vi "Offset (test).vi"(0 "RA offset":dbl format="%.2f", 1 "TCS control visa number":refnum<visa-resource-name>, 2 "TableVisaNumber":refnum<visa-resource-name>, 3 "InputVisaNumber":refnum<visa-resource-name> caption="PortNumber", 5 "DEC offset":dbl format="%.2f", 7 "Mode Offset":u32=4, 9 "Temps d'exposition":dbl=2.0 min=0.0 step=0.001 format="%.3f", 11 "Rot(rad)":dbl=3.635577729637803 format="%.2f", 12 "arcmin/pulse":dbl=5.367e-05 format="%.5e", 13 "RA Tel":dbl=45429.1344 caption="A. D." format="%<%H:%M:%S%1u>t", 14 "DEC Tel":dbl=164421.0216 caption="Déc." format="%<%H:%M:%S%0u>t") -> (8 "Undo offset":bool)   [LabVIEW 2010]
uses:
  Globals.vi
  Polymorphics/Distance(single).vi
panel:
  out "Error code":i8
  out "Guider was running":bool
  out "NewRA":dbl format="%.2f"
  out "NewDEC":dbl format="%.2f"
  out "Moffset":bool
  out "Goffset":bool=TRUE
  out "Undo startguide":bool
  in  "goto accel":u32=200 max=1000
  in  "goto vite":u32=30000 min=1 max=500000
  in  "goto lent":u32=200 min=1 max=500000
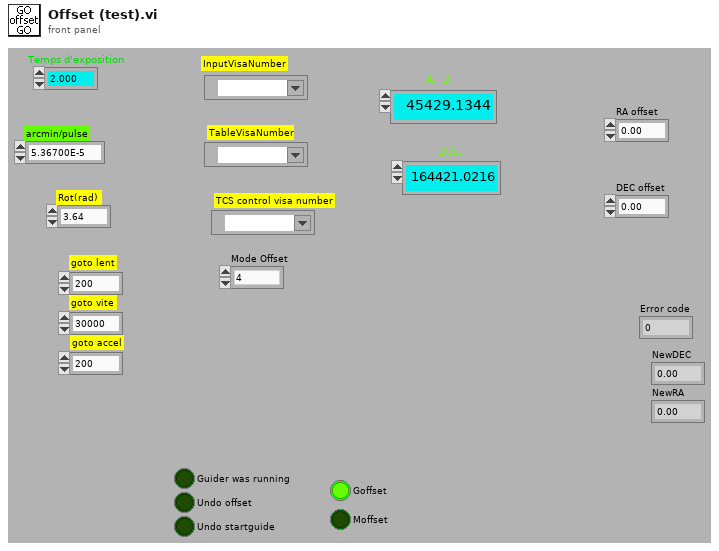
[diagram p1: front panel]
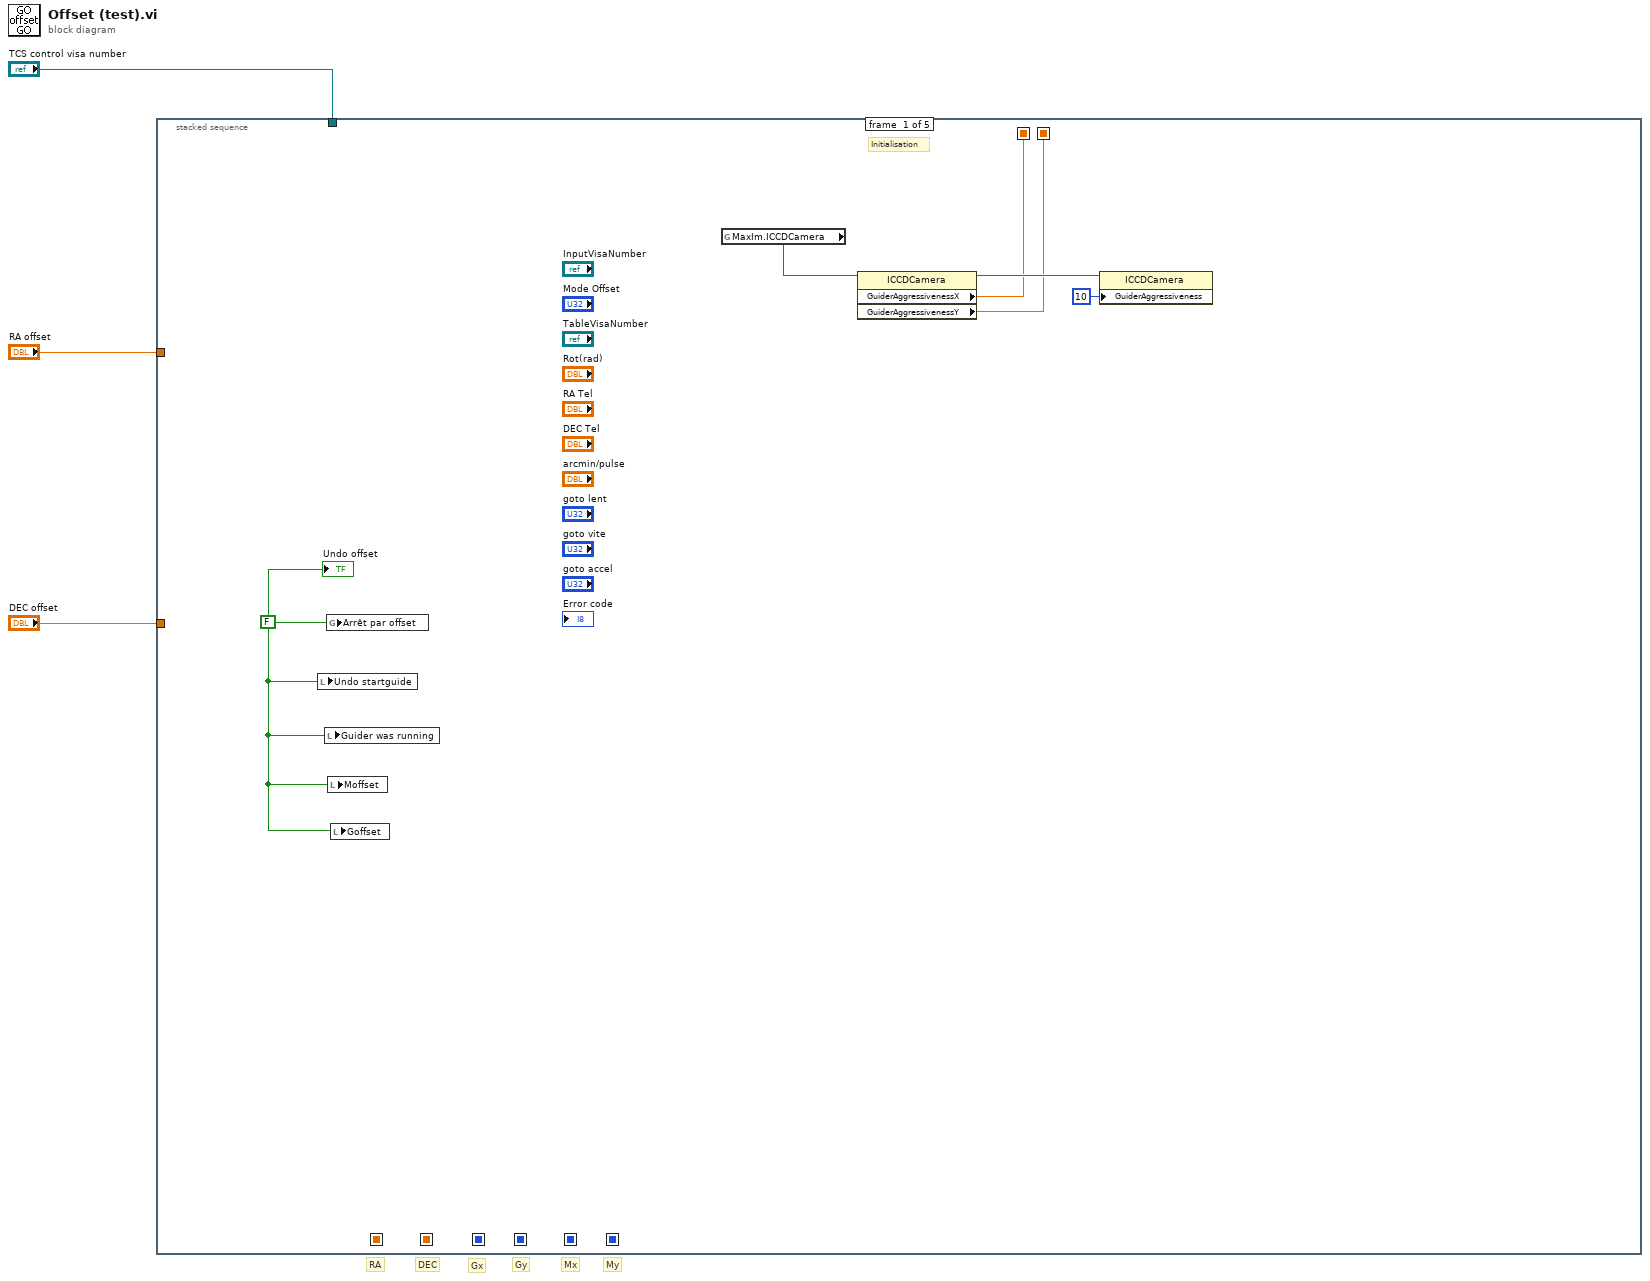
[diagram p0: block diagram]
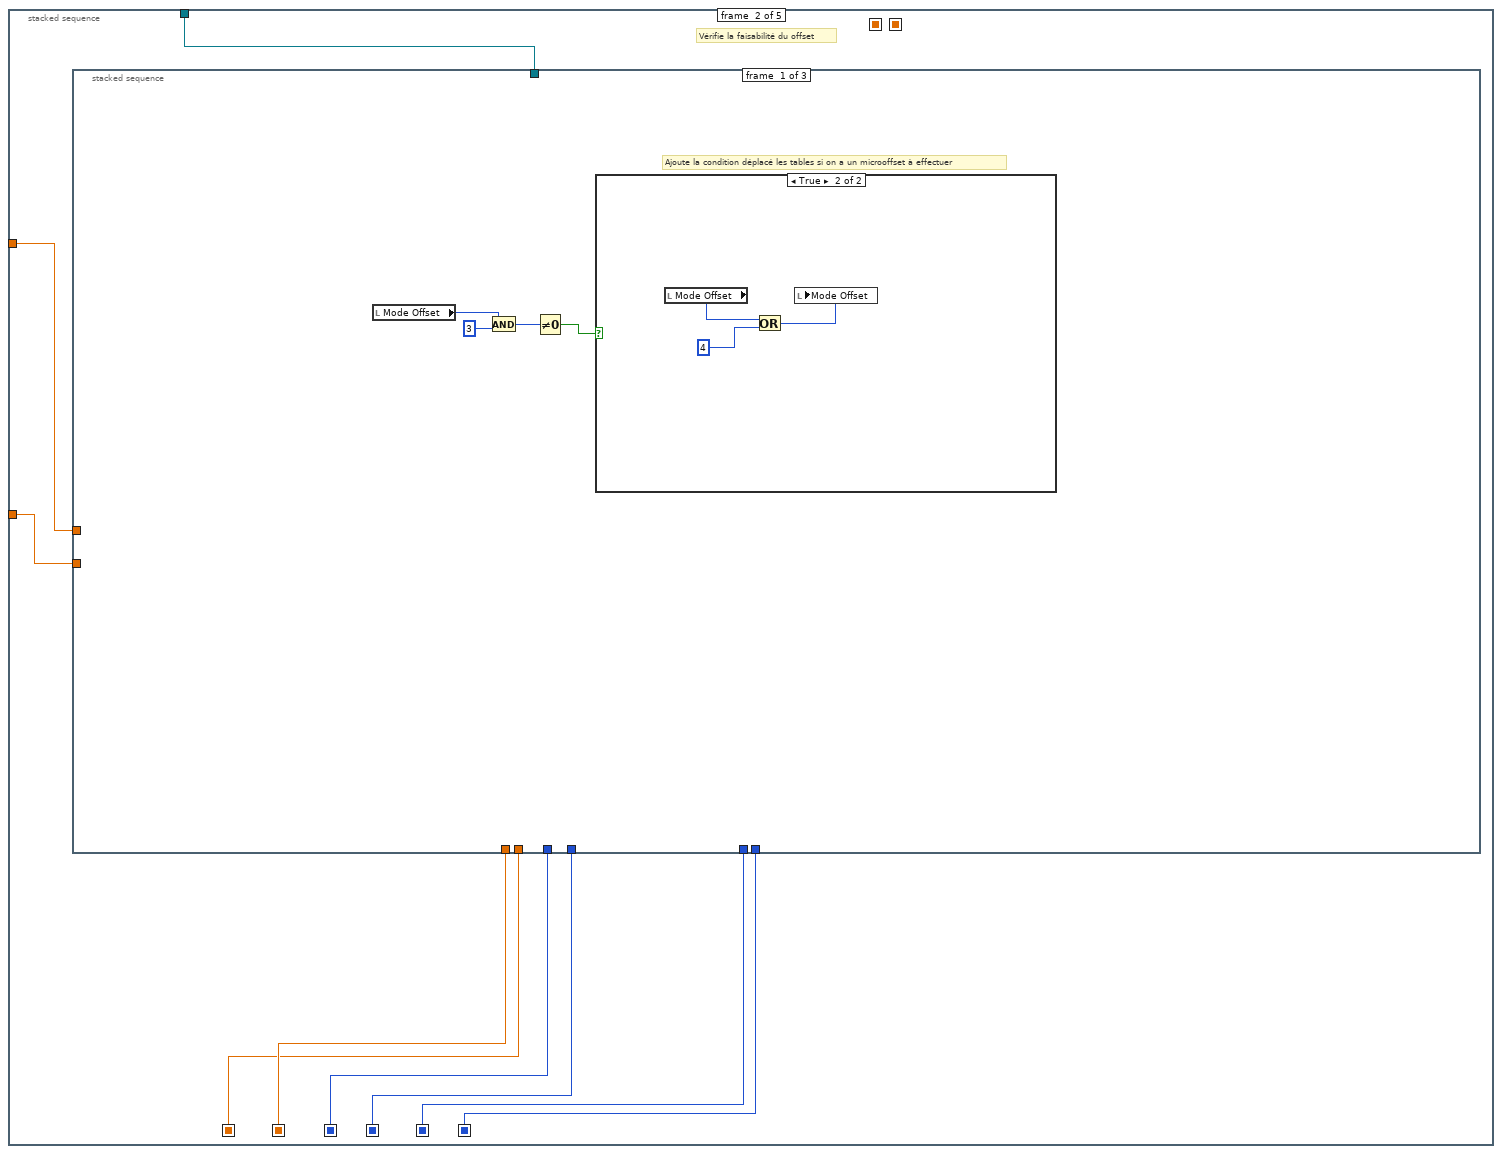
[diagram p2: hidden frame]
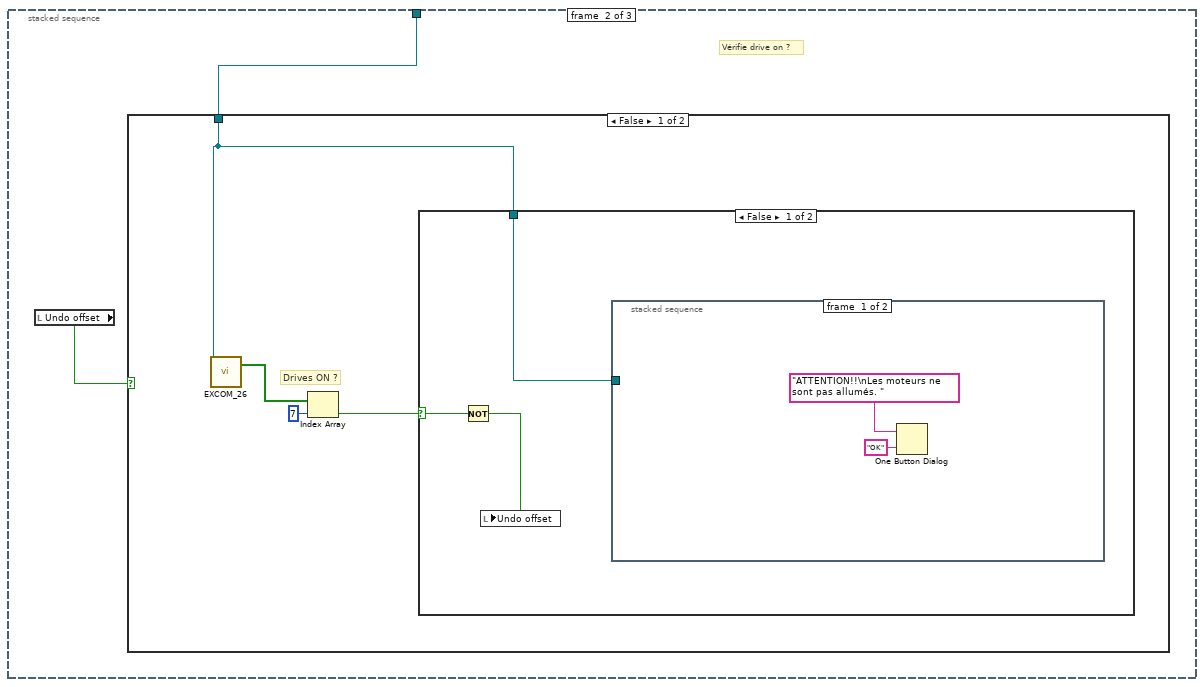
[diagram p4: hidden frame]
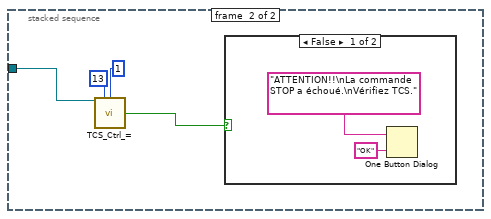
[diagram p5: hidden frame]
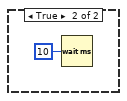
[diagram p6: hidden frame]
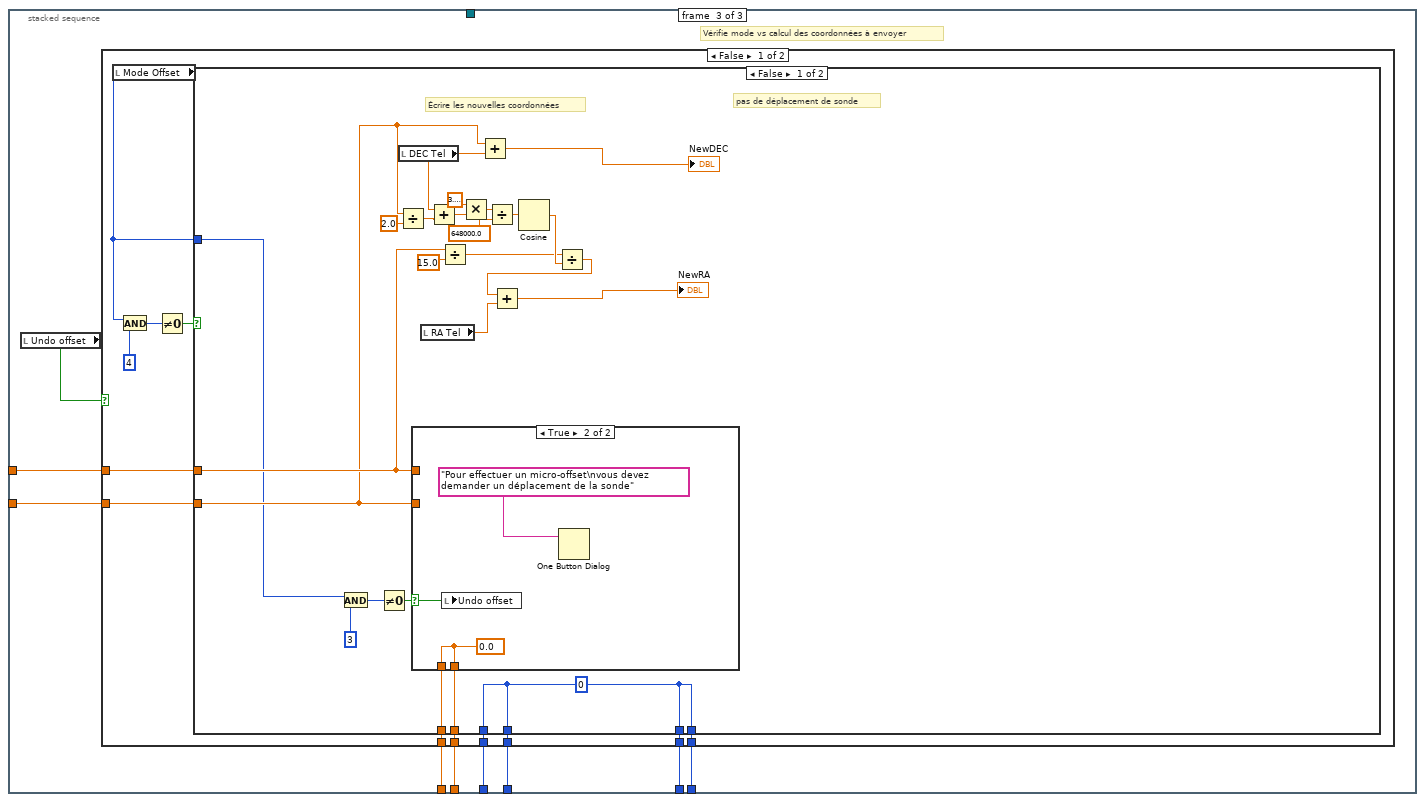
[diagram p9: hidden frame]
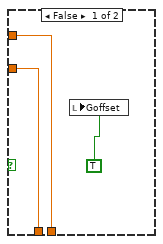
[diagram p10: hidden frame]
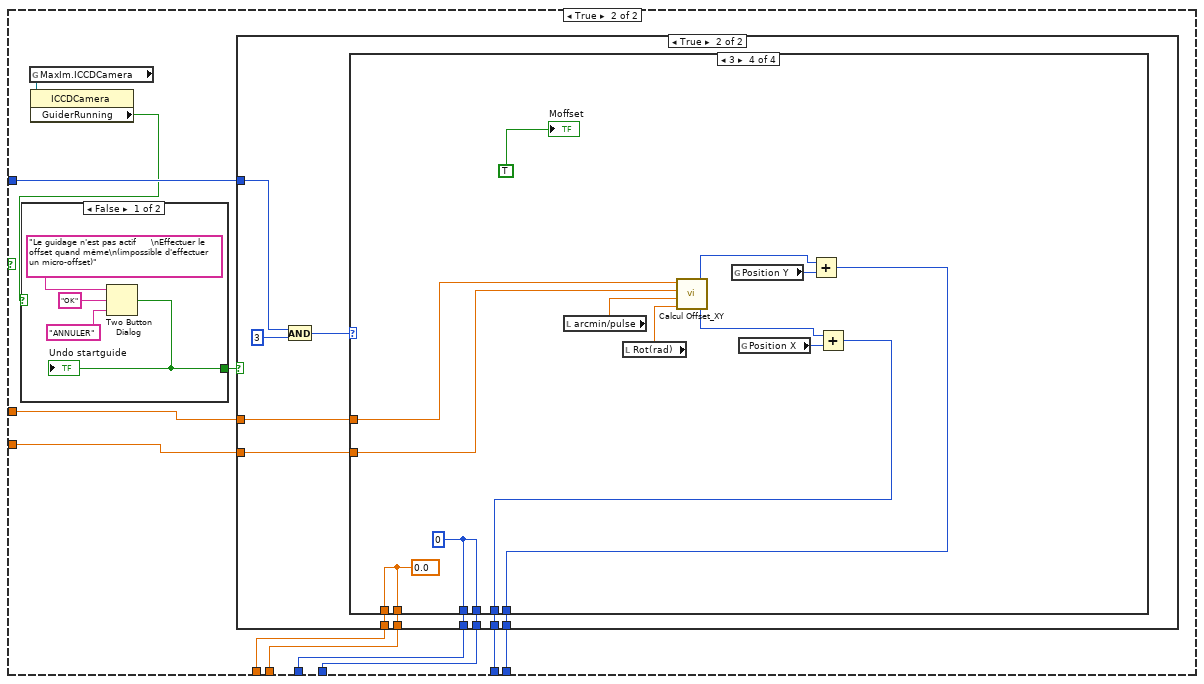
[diagram p11: hidden frame]
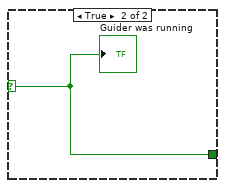
[diagram p12: hidden frame]
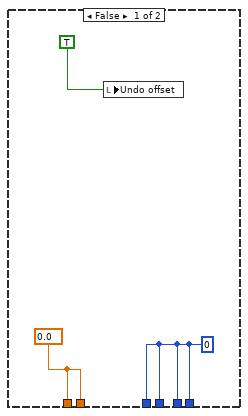
[diagram p13: hidden frame]
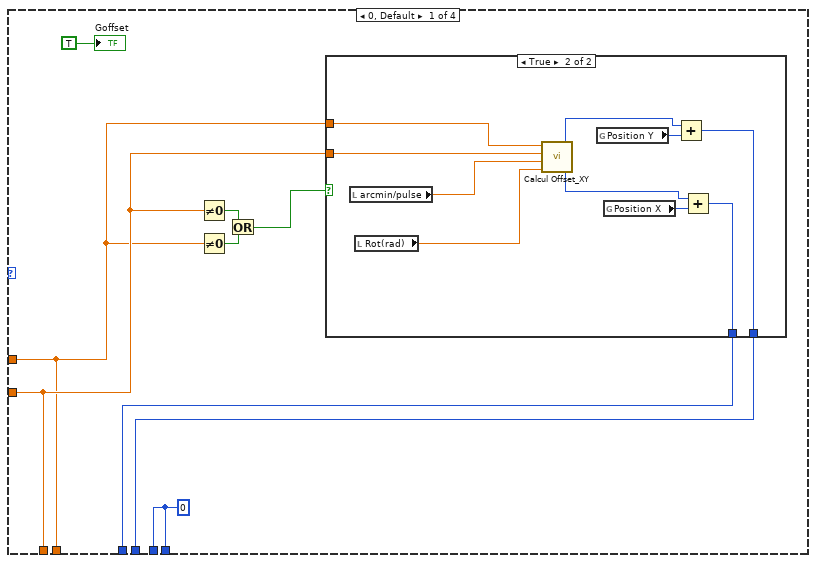
[diagram p14: hidden frame]
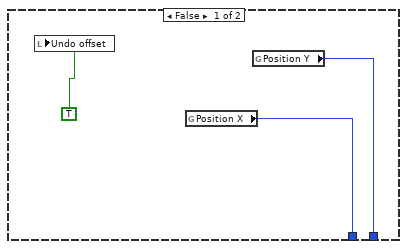
[diagram p15: hidden frame]
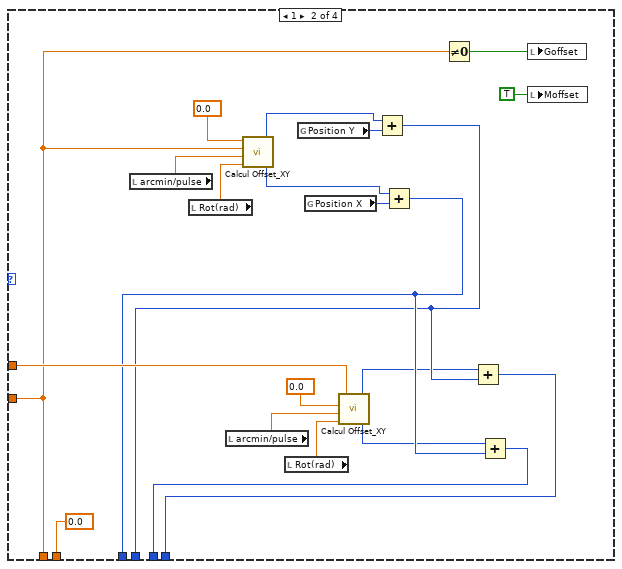
[diagram p16: hidden frame]
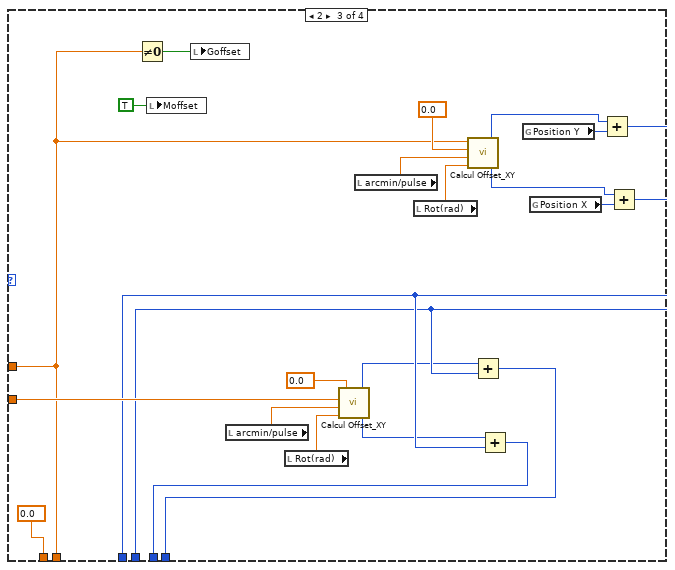
[diagram p17: hidden frame]
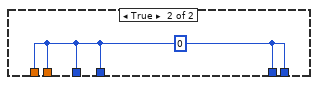
[diagram p18: hidden frame]
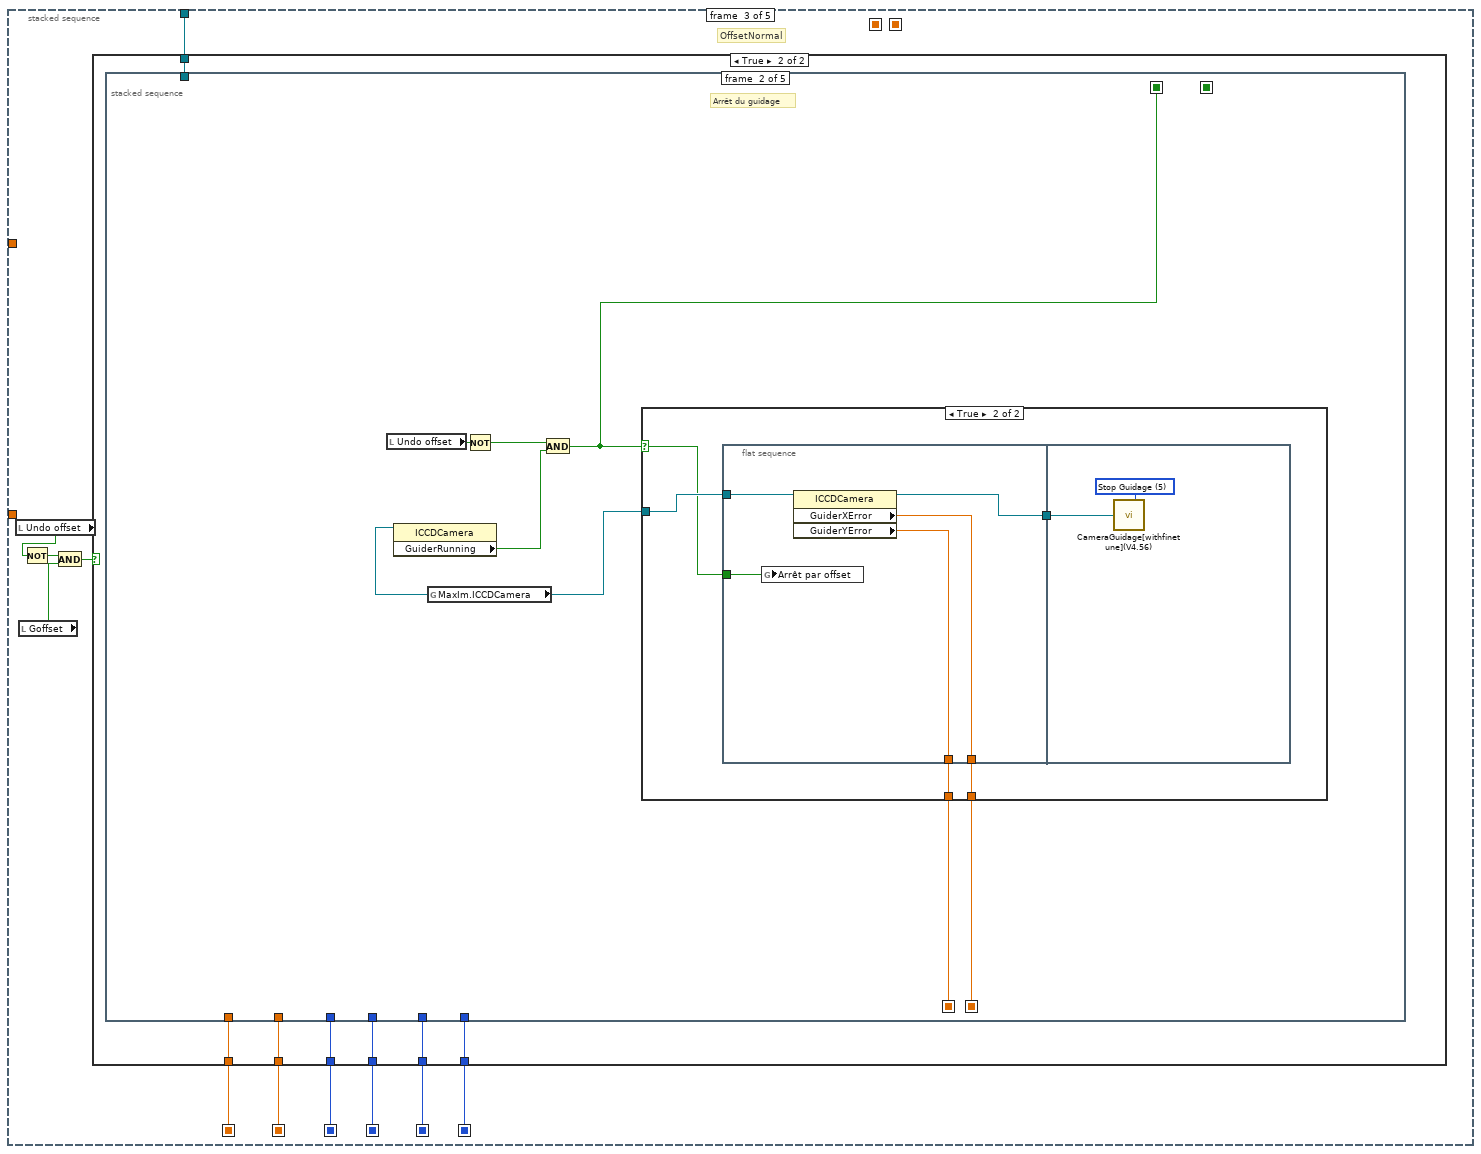
[diagram p19: hidden frame]
diagram:
  # "My"
  # "Mx"
  # "Gy"
  # "Gx"
  # "DEC"
  # "RA"
  n1 = stacked-sequence {
    seq-local: [_ w15 _ _ _] -> [_ _ w214 _ _]
    seq-local: [_ w16 _ _ _] -> [_ _ w213 _ _]
    seq-local: [_ w14 _ _ _] -> [_ _ w211 _ _]
    seq-local: [_ w13 _ _ _] -> [_ _ w210 _ _]
    seq-local: [_ w10 _ _ _] -> [_ _ w209 w444 _]
    seq-local: [_ w12 _ _ _] -> [_ _ w208 w443 _]
    seq-local: [w6 _ _ _ _] -> [_ _ _ _ w517]
    seq-local: [w5 _ _ _ _] -> [_ _ _ _ w516]
    tunnel: "DEC offset" -> [_ w17 _ _ _]
    tunnel: "RA offset" -> [_ w18 _ _ _]
    tunnel: "TCS control visa number" -> [_ w11 w212 _ _]
    frame #0 {
      w4 = FALSE
      # "Initialisation"
      n2 = local write "Undo startguide"(w4) -> ()
      n3 = local write "Guider was running"(w4) -> ()
      n4 = global write "Globals.vi" "Arrêt par offset"(w4) -> ()
      n5 = local write "Moffset"(w4) -> ()
      n6 = local write "Goffset"(w4) -> ()
      n7 = global read "Globals.vi" "MaxIm.ICCDCamera"() -> (w9:refnum<k7>)
      n8 = property class="ICCDCamera"(reference=w9) -> (reference out=w8:refnum<k7>, "GuiderAggressivenessX"=w6:sgl, "GuiderAggressivenessY"=w5:sgl)  [unwired: 1 in, 1 out]
      n9 = property class="ICCDCamera"(reference=w8, "GuiderAggressiveness"=i16 10) -> ()  [unwired: 1 in, 2 out]
      "Undo offset" <- w4
    }
    frame #1 {
      # "Vérifie la faisabilité du offset"
      n10 = stacked-sequence {
        tunnel: w11 -> [_ w27 _]
        tunnel: w18 -> [_ _ w51]
        tunnel: w17 -> [_ _ w50]
        tunnel: [_ _ w49] -> w16
        tunnel: [_ _ w48] -> w15
        tunnel: [_ _ w47] -> w14
        tunnel: [_ _ w46] -> w13
        tunnel: [_ _ w45] -> w12
        tunnel: [_ _ w44] -> w10
        frame #0 {
          # "Ajoute la condition déplacé les tables si on a un microoffset à effectuer"
          n11 = local read "Mode Offset"() -> (w22:u32)
          n12 = And(x=w22, y=u32 3) -> (x .and. y?=w20:u32)
          n13 = Not Equal To 0?(x=w20) -> (x != 0?=w19:bool)
          n14 = case shown="True" w19 {
            frame False {
            }
            frame True {
              n15 = local read "Mode Offset"() -> (w25:u32)
              n16 = Or(x=w25, y=u32 4) -> (x .or. y?=w24:u32)
              n17 = local write "Mode Offset"(w24) -> ()
            }
          }
        }
        frame #1 {
          # "Vérifie drive on ?"
          n18 = local read "Undo offset"() -> (w26:bool)
          n19 = case shown="False" w26 {
            tunnel: w27 -> [w29 _]
            frame False {
              # "Drives ON ?"
              n20 = call "EXCOM_26.vi"("VRN IN"=w29) -> ("STATH"=w30:bool[])  [unwired: 8 in, 6 out]
              n21 = Index Array(array=w30, index=7 ("Index")) -> (element=w28:bool)
              n22 = case shown="False" w28 {
                selector: w28 -> [w33 _]
                tunnel: w29 -> [w34 _]
                frame False {
                  n23 = Not(x=w33) -> (.not. x?=w32:bool)
                  n24 = local write "Undo offset"(w32) -> ()
                  n25 = stacked-sequence {
                    tunnel: w34 -> [_ w37]
                    frame #0 {
                      n26 = One Button Dialog(message="ATTENTION!!\nLes moteurs ne sont pas allumés. ", button name ("OK")="OK" ("nom du bouton (\"OK\")")) -> ()  [unwired: 1 out]
                    }
                    frame #1 {
                      n27 = call "TCS_Ctrl_=.vi"("VRN IN"=w37, "Commande #"=u16 13, "NombredArguments"=1) -> ("OK Done"=w38:bool)  [unwired: 10 in, 2 out]
                      n28 = case shown="False" w38 {
                        frame False {
                          n29 = One Button Dialog(message="ATTENTION!!\nLa commande STOP a échoué.\nVérifiez TCS.", button name ("OK")="OK" ("nom du bouton (\"OK\")")) -> ()  [unwired: 1 out]
                        }
                        frame True {
                          n30 = Wait (ms)(milliseconds to wait=u32 10 ("attente (ms)")) -> ()  [unwired: 1 out]
                        }
                      }
                    }
                  }
                }
                frame True {
                }
              }
            }
            frame True {
            }
          }
        }
        frame #2 {
          # "Vérifie mode vs calcul des coordonnées à envoyer"
          n31 = local read "Undo offset"() -> (w52:bool)
          n32 = case shown="False" w52 {
            tunnel: w51 -> [w60 _]
            tunnel: w50 -> [w59 _]
            tunnel: [w58 w203] -> w49
            tunnel: [w57 w203] -> w48
            tunnel: [w56 w203] -> w47
            tunnel: [w55 w203] -> w46
            tunnel: [w54 w203] -> w44
            tunnel: [w53 w203] -> w45
            frame False {
              n33 = local read "Mode Offset"() -> (w61:u32)
              n34 = And(x=w61, y=u32 4) -> (x .and. y?=w63:u32)
              n35 = Not Equal To 0?(x=w63) -> (x != 0?=w62:bool)
              n36 = case shown="False" w62 {
                tunnel: w61 -> [w67 w106]
                tunnel: w60 -> [w74 w102]
                tunnel: w59 -> [w73 w103]
                tunnel: [w72 w105] -> w58
                tunnel: [w71 w104] -> w57
                tunnel: [w75 w101] -> w56
                tunnel: [w75 w100] -> w55
                tunnel: [w75 w96] -> w54
                tunnel: [w75 w95] -> w53
                frame False {
                  w75 = 0
                  # "Écrire les nouvelles coordonnées"
                  # "pas de déplacement de sonde"
                  n37 = And(x=w67, y=u32 3) -> (x .and. y?=w70:u32)
                  n38 = Not Equal To 0?(x=w70) -> (x != 0?=w68:bool)
                  n39 = Divide(x=w73, y=2.0) -> (x/y=w80:dbl)
                  n40 = local read "DEC Tel"() -> (w77:dbl)
                  n41 = case shown="True" w68 {
                    selector: w68 -> [_ w93]
                    tunnel: w74 -> [w90 _]
                    tunnel: w73 -> [w91 _]
                    tunnel: [w91 w94] -> w72
                    tunnel: [w90 w94] -> w71
                    frame False {
                      n42 = local write "Goffset"(TRUE) -> ()
                    }
                    frame True {
                      w94 = 0.0 ("Offset Déc")
                      n43 = local write "Undo offset"(w93) -> ()
                      n44 = One Button Dialog(message="Pour effectuer un micro-offset\nvous devez demander un déplacement de la sonde") -> ()  [unwired: 1 in, 1 out]
                    }
                  }
                  n45 = local read "RA Tel"() -> (w76:dbl)
                  n46 = Add(x=w77, y=w80) -> (x+y=w81:dbl)
                  n47 = Divide(x=w74, y=15.0) -> (x/y=w86:dbl)
                  n48 = Multiply(x=3.141592653589793, y=w81) -> (x*y=w83:dbl)
                  n49 = Add(x=w73, y=w77) -> (x+y=→"NewDEC":dbl)
                  n50 = Divide(x=w83, y=648000.0) -> (x/y=w85:dbl)
                  n51 = Cosine(x=w85) -> (cos(x)=w87:dbl)
                  n52 = Divide(x=w86, y=w87) -> (x/y=w88:dbl)
                  n53 = Add(x=w88, y=w76) -> (x+y=→"NewRA":dbl)
                }
                frame True {
                  n54 = global read "Globals.vi" "MaxIm.ICCDCamera"() -> (w99:refnum<k7>)
                  n55 = property class="ICCDCamera"(reference=w99) -> ("GuiderRunning"=w98:bool)  [unwired: 1 in, 2 out]
                  n56 = case shown="False" w98 {
                    selector: w98 -> [_ w111]
                    tunnel: [w107 w111] -> w97
                    frame False {
                      n57 = Two Button Dialog(message="Le guidage n'est pas actif     \nEffectuer le offset quand même\n(impossible d'effectuer un micro-offset)", 1:"ANNULER" ("Nom du bouton F (\"Annuler\")"), 2:"OK" ("Nom du bouton V (\"OK\")")) -> (T button?=w107:bool)
                      "Undo startguide" <- w107
                    }
                    frame True {
                      "Guider was running" <- w111
                    }
                  }
                  n58 = case shown="True" w97 {
                    tunnel: w106 -> [_ w117]
                    tunnel: [w114 w125] -> w105
                    tunnel: [w114 w124] -> w104
                    tunnel: w103 -> [_ w123]
                    tunnel: w102 -> [_ w122]
                    tunnel: [w112 w121] -> w101
                    tunnel: [w112 w120] -> w100
                    tunnel: [w112 w119] -> w96
                    tunnel: [w112 w118] -> w95
                    frame False {
                      w112 = 0
                      w114 = 0.0 ("Offset Déc")
                      n59 = local write "Undo offset"(TRUE) -> ()
                    }
                    frame True {
                      n60 = And(x=w117, y=u32 3) -> (x .and. y?=w115:u32)
                      n61 = case shown="3" w115 {
                        tunnel: [w127 w153 0.0 ("Offset A.D.") w202] -> w125
                        tunnel: [w126 0.0 ("Offset A.D.") w174 w202] -> w124
                        tunnel: w123 -> [w127 w153 w177 w195]
                        tunnel: w122 -> [w126 w157 w174 w196]
                        tunnel: [w132 w151 w172 w201] -> w121
                        tunnel: [w131 w150 w171 w201] -> w120
                        tunnel: [w134 w158 w180 w192] -> w119
                        tunnel: [w134 w159 w181 w193] -> w118
                        frame 0, Default {
                          w134 = 0
                          n62 = Not Equal To 0?(x=w127) -> (x != 0?=w130:bool)
                          n63 = Not Equal To 0?(x=w126) -> (x != 0?=w129:bool)
                          n64 = Or(x=w130, y=w129) -> (x .or. y?=w128:bool)
                          n65 = case shown="True" w128 {
                            tunnel: w126 -> [_ w147]
                            tunnel: w127 -> [_ w146]
                            tunnel: [w135 w139] -> w132
                            tunnel: [w136 w138] -> w131
                            frame False {
                              n66 = local write "Undo offset"(TRUE) -> ()
                              n67 = global read "Globals.vi" "Position X"() -> (w135:i32)
                              n68 = global read "Globals.vi" "Position Y"() -> (w136:i32)
                            }
                            frame True {
                              n69 = local read "arcmin/pulse"() -> (w140:dbl)
                              n70 = local read "Rot(rad)"() -> (w141:dbl)
                              n71 = call "Calcul Offset_XY.vi"("Rot(rad)"=w141, "Arcmin/pulse"=w140, "offset DEC"=w146, "offset RA"=w147) -> ("X"=w142:i32, "Y"=w143:i32)
                              n72 = global read "Globals.vi" "Position Y"() -> (w145:i32)
                              n73 = global read "Globals.vi" "Position X"() -> (w144:i32)
                              n74 = Add(x=w143, y=w145) -> (x+y=w138:i32)
                              n75 = Add(x=w142, y=w144) -> (x+y=w139:i32)
                            }
                          }
                          "Goffset" <- TRUE
                        }
                        frame 1 {
                          n76 = local read "arcmin/pulse"() -> (w167:dbl)
                          n77 = local read "Rot(rad)"() -> (w166:dbl)
                          n78 = local read "arcmin/pulse"() -> (w160:dbl)
                          n79 = call "Calcul Offset_XY.vi"("Rot(rad)"=w166, "Arcmin/pulse"=w167, "offset DEC"=w153, "offset RA"=0.0 ("Offset A.D.")) -> ("X"=w165:i32, "Y"=w164:i32)
                          n80 = local read "Rot(rad)"() -> (w161:dbl)
                          n81 = global read "Globals.vi" "Position Y"() -> (w162:i32)
                          n82 = global read "Globals.vi" "Position X"() -> (w163:i32)
                          n83 = call "Calcul Offset_XY.vi"("Rot(rad)"=w161, "Arcmin/pulse"=w160, "offset DEC"=0.0 ("Offset A.D."), "offset RA"=w157) -> ("X"=w149:i32, "Y"=w148:i32)
                          n84 = Add(x=w164, y=w162) -> (x+y=w150:i32)
                          n85 = Add(x=w165, y=w163) -> (x+y=w151:i32)
                          n86 = Not Equal To 0?(x=w153) -> (x != 0?=w152:bool)
                          n87 = Add(x=w148, y=w150) -> (x+y=w159:i32)
                          n88 = Add(x=w149, y=w151) -> (x+y=w158:i32)
                          n89 = local write "Goffset"(w152) -> ()
                          n90 = local write "Moffset"(TRUE) -> ()
                        }
                        frame 2 {
                          n91 = Not Equal To 0?(x=w174) -> (x != 0?=w173:bool)
                          n92 = local write "Moffset"(TRUE) -> ()
                          n93 = local write "Goffset"(w173) -> ()
                          n94 = local read "arcmin/pulse"() -> (w182:dbl)
                          n95 = local read "Rot(rad)"() -> (w183:dbl)
                          n96 = call "Calcul Offset_XY.vi"("Rot(rad)"=w183, "Arcmin/pulse"=w182, "offset DEC"=w177, "offset RA"=0.0 ("Offset A.D.")) -> ("X"=w169:i32, "Y"=w170:i32)
                          n97 = local read "arcmin/pulse"() -> (w189:dbl)
                          n98 = local read "Rot(rad)"() -> (w188:dbl)
                          n99 = call "Calcul Offset_XY.vi"("Rot(rad)"=w188, "Arcmin/pulse"=w189, "offset DEC"=0.0 ("Offset A.D."), "offset RA"=w174) -> ("X"=w187:i32, "Y"=w186:i32)
                          n100 = global read "Globals.vi" "Position Y"() -> (w184:i32)
                          n101 = global read "Globals.vi" "Position X"() -> (w185:i32)
                          n102 = Add(x=w186, y=w184) -> (x+y=w171:i32)
                          n103 = Add(x=w170, y=w171) -> (x+y=w181:i32)
                          n104 = Add(x=w187, y=w185) -> (x+y=w172:i32)
                          n105 = Add(x=w169, y=w172) -> (x+y=w180:i32)
                        }
                        frame 3 {
                          w201 = 0
                          w202 = 0.0
                          n106 = local read "arcmin/pulse"() -> (w200:dbl)
                          n107 = local read "Rot(rad)"() -> (w199:dbl)
                          n108 = call "Calcul Offset_XY.vi"("Rot(rad)"=w199, "Arcmin/pulse"=w200, "offset DEC"=w195, "offset RA"=w196) -> ("X"=w191:i32, "Y"=w190:i32)
                          n109 = global read "Globals.vi" "Position Y"() -> (w197:i32)
                          n110 = global read "Globals.vi" "Position X"() -> (w198:i32)
                          n111 = Add(x=w190, y=w197) -> (x+y=w193:i32)
                          n112 = Add(x=w191, y=w198) -> (x+y=w192:i32)
                          "Moffset" <- TRUE
                        }
                      }
                    }
                  }
                }
              }
            }
            frame True {
              w203 = 0
            }
          }
        }
      }
    }
    frame #2 {
      # "OffsetNormal"
      n113 = local read "Undo offset"() -> (w205:bool)
      n114 = local read "Goffset"() -> (w204:bool)
      n115 = Not(x=w205) -> (.not. x?=w206:bool)
      n116 = And(x=w206, y=w204) -> (x .and. y?=w207:bool)
      n117 = case shown="True" w207 {
        tunnel: w214 -> [_ w221]
        tunnel: w213 -> [_ w220]
        tunnel: w212 -> [_ w219]
        tunnel: w211 -> [_ w218]
        tunnel: w210 -> [_ w217]
        tunnel: w209 -> [_ w216]
        tunnel: w208 -> [_ w215]
        frame False {
        }
        frame True {
          n118 = stacked-sequence {
            seq-local: [_ w253 _ _ _] -> [_ _ _ w382 _]
            seq-local: [_ _ _ w381 _] -> [_ _ _ _ w401]
            seq-local: [_ w254 _ _ _] -> [_ _ _ _ w399]
            seq-local: [_ w255 _ _ _] -> [_ _ _ _ w398]
            tunnel: w221 -> [w223 _ _ _ _]
            tunnel: w220 -> [w222 _ _ _ _]
            tunnel: w219 -> [w227 _ w273 _ _]
            tunnel: w218 -> [_ _ w278 _ _]
            tunnel: w217 -> [_ _ w277 _ _]
            tunnel: w216 -> [_ _ w276 _ _]
            tunnel: w215 -> [_ _ w275 _ _]
            frame #0 {
              # "Envoie de la commande de offset"
              n119 = call "TCS_Ctrl_=.vi"("VRN IN"=w227, "Commande #"=u16 7, "NombredArguments"=3, "string1"=w223, "string2"=w222) -> ("OK Done"=w224:bool)  [unwired: 8 in, 2 out]
              n120 = case shown="True" w224 {
                tunnel: w227 -> [_ w231]
                frame False {
                  n121 = local write "Undo offset"(TRUE) -> ()
                  n122 = One Button Dialog(message="ATTENTION!!\nLa commande OFFSET a échoué.\nVérifiez TCS.", button name ("OK")="OK" ("nom du bouton (\"OK\")")) -> ()  [unwired: 1 out]
                }
                frame True {
                  n123 = while {
                    tunnel: [w246] -> w232
                    tunnel: w231 -> [w243]
                    stop <- w248 stop-if-true
                    n124 = call "EXCOM_26.vi"("VRN IN"=w243) -> ("STATL"=w245:bool[], "STATH"=w244:bool[])  [unwired: 8 in, 5 out]
                    n125 = Index Array(array=w245, index=3 ("Index")) -> (element=w246:bool)
                    n126 = Index Array(array=w244, index=4 ("Index")) -> (element=w242:bool)
                    n127 = case shown="False" w242 {
                      selector: w242 -> [_ w252]
                      frame False {
                      }
                      frame True {
                        n128 = local write "Undo offset"(w252) -> ()
                        n129 = One Button Dialog(message="La position cible est inaccessible\n             offset annulé") -> ()  [unwired: 1 in, 1 out]
                      }
                    }
                    n130 = Or(x=w246, y=w242) -> (x .or. y?=w248:bool)
                    n131 = Wait Until Next ms Multiple(millisecond multiple=u32 100 ("n millisecondes")) -> ()  [unwired: 1 out]
                  }
                  n132 = case shown="False" w232 {
                    tunnel: w231 -> [w234 _]
                    frame False {
                      n133 = One Button Dialog(message="ATTENTION !!\nLes coordonées de la cible\nne peuvent être atteintes.\nAnnulez la commande.", button name ("OK")="OK" ("nom du bouton (\"OK\")")) -> ()  [unwired: 1 out]
                      n134 = call "TCS_Ctrl_=.vi"("VRN IN"=w234, "Commande #"=u16 13, "NombredArguments"=1) -> ("OK Done"=w233:bool)  [unwired: 10 in, 2 out]
                      n135 = case shown="False" w233 {
                        frame False {
                          n136 = One Button Dialog(message="ATTENTION!!\nLa commande STOP a échoué.\nVérifiez TCS.", button name ("OK")="OK" ("nom du bouton (\"OK\")")) -> ()  [unwired: 1 out]
                        }
                        frame True {
                          n137 = Wait (ms)(milliseconds to wait=u32 10 ("attente (ms)")) -> ()  [unwired: 1 out]
                        }
                      }
                    }
                    frame True {
                    }
                  }
                }
              }
            }
            frame #1 {
              # "Arrêt du guidage"
              n138 = local read "Undo offset"() -> (w257:bool)
              n139 = global read "Globals.vi" "MaxIm.ICCDCamera"() -> (w258:refnum<k7>)
              n140 = property class="ICCDCamera"(reference=w258) -> ("GuiderRunning"=w259:bool)  [unwired: 1 in, 2 out]
              n141 = Not(x=w257) -> (.not. x?=w256:bool)
              n142 = And(x=w256, y=w259) -> (x .and. y?=w253:bool)
              n143 = case shown="True" w253 {
                selector: w253 -> [_ w261]
                tunnel: w258 -> [_ w265]
                tunnel: [w260 w263] -> w255
                tunnel: [w260 w262] -> w254
                frame False {
                  w260 = sgl 0.0 ("GuiderYError")
                }
                frame True {
                  n144 = flat-sequence {
                    tunnel: w265 -> [w270]
                    tunnel: [w269] -> w264
                    tunnel: [w268] -> w263
                    tunnel: [w267] -> w262
                    tunnel: w261 -> [w266]
                    tunnel: w264 -> [w271]
                    frame #0 {
                      n145 = global write "Globals.vi" "Arrêt par offset"(w266) -> ()
                      n146 = property class="ICCDCamera"(reference=w270) -> (reference out=w269:refnum<k7>, "GuiderXError"=w268:sgl, "GuiderYError"=w267:sgl)  [unwired: 1 in, 1 out]
                    }
                    frame #1 {
                      w272 = u16 5 items=["Exposition Guideur", "Calibration", "Guidage", "Piedestal", "Exposition simple", "Stop Guidage"] ("Mode")
                      n147 = call "CameraGuidage[withfinetune](V4.56).vi"("Mode"=w272, "MaxIm.ICCDCamera"=w271) -> ()  [unwired: 11 in, 3 out]
                    }
                  }
                }
              }
            }
            frame #2 {
              # "Envoie des commandes de déplacements"
              n148 = local read "Undo offset"() -> (w274:bool)
              n149 = case shown="False" w274 {
                tunnel: w278 -> [w280 _]
                tunnel: w277 -> [w279 _]
                tunnel: w276 -> [w286 _]
                tunnel: w275 -> [w285 _]
                tunnel: w273 -> [w281 _]
                frame False {
                  w287 = 1000000
                  w290 = 0
                  w291 = 0
                  w294 = 1000000
                  n150 = In Range and Coerce(upper limit=w294, x=w280, lower limit=w291) -> (In Range?=w292:bool)  [unwired: 1 out]
                  n151 = In Range and Coerce(upper limit=w294, x=w279, lower limit=w291) -> (In Range?=w293:bool)  [unwired: 1 out]
                  n152 = In Range and Coerce(upper limit=w287, x=w286, lower limit=w290) -> (In Range?=w289:bool)  [unwired: 1 out]
                  n153 = In Range and Coerce(upper limit=w287, x=w285, lower limit=w290) -> (In Range?=w288:bool)  [unwired: 1 out]
                  n154 = And(x=w292, y=w293) -> (x .and. y?=w283:bool)
                  n155 = And(x=w289, y=w288) -> (x .and. y?=w284:bool)
                  n156 = Or(x=w283, y=w284) -> (x .or. y?=w282:bool)
                  n157 = case shown="True" w282 {
                    tunnel: w281 -> [_ w309]
                    tunnel: w280 -> [_ w301]
                    tunnel: w279 -> [_ w300]
                    frame False {
                      n158 = local write "Undo offset"(TRUE) -> ()
                      n159 = Two Button Dialog(message="La position de la sonde\nne pourra être restaurée\naprès le déplacement par offset.", 1:"Annuler" ("Nom du bouton V (\"OK\")"), 2:"OK" ("Nom du bouton V (\"OK\")")) -> ()  [unwired: 1 out]
                    }
                    frame True {
                      # "Déplacer le\n télescope"
                      n160 = global write "Globals.vi" "Moniteur table"(TRUE ("Direction")) -> ()
                      n161 = local read "Mode Offset"() -> (w305:u32)
                      n162 = local read "TableVisaNumber"() -> (w308:refnum<visa-resource-name>)
                      n163 = And(x=w305, y=u32 4) -> (x .and. y?=w303:u32)
                      n164 = Not Equal To 0?(x=w303) -> (x != 0?=w302:bool)
                      n165 = call "TCS_Ctrl_=.vi"("VRN IN"=w309, "Commande #"=u16 12, "NombredArguments"=1) -> ("OK Done"=w306:bool)  [unwired: 10 in, 2 out]
                      n166 = And(x=w306, y=w302) -> (x .and. y?=w307:bool)
                      n167 = case shown="True" w307 {
                        tunnel: w300 -> [_ w313]
                        tunnel: w301 -> [_ w315]
                        tunnel: w308 -> [_ w321]
                        frame False {
                        }
                        frame True {
                          # "Déplacer la sonde"
                          n168 = while {
                            tunnel: w315 -> [w324]
                            tunnel: [w324] -> w314
                            tunnel: w313 -> [w323]
                            tunnel: [w323] -> w312
                            i -> [w330]
                            stop <- w328 stop-if-true
                            n169 = global read "Globals.vi" "Busy"() -> (w326:bool)
                            n170 = Wait (ms)(milliseconds to wait=u32 100) -> ()  [unwired: 1 out]
                            n171 = Not(x=w326) -> (.not. x?=w325:bool)
                            n172 = call "max-iteration.vi"("i max"=10, "i act"=w330, "Valeur entrante"=w325) -> ("break ?"=w328:bool)
                          }
                          n173 = global read "Globals.vi" "Position Z"() -> (w317:i32)
                          n174 = global read "Globals.vi" "Position P"() -> (w316:i32)
                          n175 = global write "Globals.vi" "CibleX"(w314) -> ()
                          n176 = global write "Globals.vi" "CibleY"(w312) -> ()
                          n177 = local read "goto lent"() -> (w320:u32)
                          n178 = local read "goto accel"() -> (w319:u32)
                          n179 = local read "goto vite"() -> (w318:u32)
                          n180 = while {
                            tunnel: w320 -> [w340]
                            tunnel: w319 -> [w339]
                            tunnel: w318 -> [w338]
                            tunnel: w312 -> [w337]
                            tunnel: w314 -> [w336]
                            tunnel: w316 -> [w335]
                            tunnel: w317 -> [w334]
                            tunnel: w321 -> [w333]
                            tunnel: [w331] -> w322
                            i -> [w343]
                            stop <- w332 stop-if-true
                            n181 = call "GotoTables(aligned).vi"("High Speed"=w338, "Acceleration Time"=w339, "Low Speed"=w340, "VISA resource name"=w333, "Pulse P"=w335, "Pulse Z"=w334, "Pulse X"=w336, "Pulse Y"=w337) -> ("OK Done"=w331:bool)
                            n182 = call "max-iteration.vi"("i max"=10, "i act"=w343, "Valeur entrante"=w331) -> ("break ?"=w332:bool)
                            n183 = Wait Until Next ms Multiple(millisecond multiple=u32 200) -> ()  [unwired: 1 out]
                          }
                          n184 = case shown="False" w322 {
                            selector: w322 -> [w344 _]
                            frame False {
                              n185 = global write "Globals.vi" "Moniteur table"(w344) -> ()
                              n186 = local write "Undo offset"(TRUE) -> ()
                              n187 = One Button Dialog(message="ATTENTION!!\nLa commande de déplacement\ndes tables a échoué.\nVérifiez le contrôleur des tables.", button name ("OK")="OK" ("nom du bouton (\"OK\")")) -> ()  [unwired: 1 out]
                            }
                            frame True {
                            }
                          }
                        }
                      }
                      n188 = case shown="True" w306 {
                        tunnel: w309 -> [_ w351]
                        frame False {
                          n189 = local write "Undo offset"(TRUE) -> ()
                          n190 = One Button Dialog(message="ATTENTION!!\nProblème de communication\navec TCS-Ctrl", button name ("OK")="OK" ("nom du bouton (\"OK\")")) -> ()  [unwired: 1 out]
                        }
                        frame True {
                          n191 = stacked-sequence {
                            tunnel: w351 -> [_ w353]
                            frame #0 {
                              # "Attendre 500ms que la commande GO soit acceptée"
                              n192 = Wait (ms)(milliseconds to wait=u32 500 ("attente (ms)")) -> ()  [unwired: 1 out]
                            }
                            frame #1 {
                              n193 = Tick Count (ms)() -> (millisecond timer value=w355:u32)
                              n194 = while {
                                tunnel: w355 -> [w376]
                                tunnel: [w373] -> w354
                                tunnel: w353 -> [w368]
                                stop <- w375 stop-if-true
                                # "Max 90 secondes"
                                # "Bit 7 = slew ON ou OFF"
                                n195 = Tick Count (ms)() -> (millisecond timer value=w377:u32)
                                n196 = call "EXCOM_26.vi"("VRN IN"=w368) -> ("STATL"=w369:bool[])  [unwired: 8 in, 6 out]
                                n197 = Subtract(x=w377, y=w376) -> (x-y=w378:u32)
                                n198 = Greater?(x=w378, y=u32 90000) -> (0:w373:bool)
                                n199 = Index Array(array=w369, index=7 ("Index")) -> (element=w370:bool)
                                n200 = Not(x=w370) -> (.not. x?=w372:bool)
                                n201 = Or(x=w372, y=w373) -> (x .or. y?=w375:bool)
                                n202 = Wait Until Next ms Multiple(millisecond multiple=u32 500 ("n millisecondes")) -> ()  [unwired: 1 out]
                              }
                              n203 = case shown="True" w354 {
                                tunnel: w353 -> [_ w357]
                                frame False {
                                }
                                frame True {
                                # "timeout"
                                n204 = local write "Undo offset"(TRUE) -> ()
                                n205 = One Button Dialog(message="ATTENTION!!\nProblème de déplacement\ndu télescope.", button name ("OK")="OK" ("nom du bouton (\"OK\")")) -> (true=w358:bool)
                                n206 = case shown="True" w358 {
                                tunnel: w357 -> [_ w361]
                                frame False {
                                }
                                frame True {
                                n207 = call "TCS_Ctrl_=.vi"("VRN IN"=w361, "Commande #"=u16 13, "NombredArguments"=1) -> ("OK Done"=w362:bool)  [unwired: 10 in, 2 out]
                                n208 = case shown="False" w362 {
                                frame False {
                                n209 = One Button Dialog(message="ATTENTION!!\nLa commande STOP a échoué.\nVérifiez TCS.", button name ("OK")="OK" ("nom du bouton (\"OK\")")) -> ()  [unwired: 1 out]
                                }
                                frame True {
                                n210 = Wait (ms)(milliseconds to wait=u32 10 ("attente (ms)")) -> ()  [unwired: 1 out]
                                }
                                }
                                }
                                }
                                }
                              }
                            }
                          }
                        }
                      }
                    }
                  }
                }
                frame True {
                }
              }
            }
            frame #3 {
              # "Vérifie que le offset est complété et\nredémarre le guidage"
              n211 = local read "Undo offset"() -> (w380:bool)
              n212 = case shown="False" w380 {
                tunnel: w382 -> [w388 _]
                tunnel: [w387 FALSE] -> w381
                frame False {
                  n213 = local read "Mode Offset"() -> (w386:u32)
                  n214 = And(x=w386, y=u32 4) -> (x .and. y?=w384:u32)
                  n215 = Equal To 0?(x=w384) -> (x = 0?=w383:bool)
                  n216 = case shown="False" w383 {
                    tunnel: w388 -> [w391 _]
                    tunnel: [w389 FALSE] -> w387
                    frame False {
                      # "Vérifier si la sonde a atteint la nouvelle position\nRedémarrer le guidage automatique si nécessaire"
                      n217 = while {
                        tunnel: [w393] -> w392
                        stop <- w393 stop-if-true
                        n218 = global read "Globals.vi" "Moniteur table"() -> (w394:bool)
                        n219 = Wait Until Next ms Multiple(millisecond multiple=u32 200 ("n millisecondes")) -> ()  [unwired: 1 out]
                        n220 = Not(x=w394) -> (.not. x?=w393:bool)
                      }
                      n221 = local read "Undo startguide"() -> (w390:bool)
                      n222 = Compound Arithmetic op=AND(w391, w392, invert w390) -> (w389:bool)
                      n223 = global write "Globals.vi" "StartGuide"(w389) -> ()
                    }
                    frame True {
                    }
                  }
                }
                frame True {
                }
              }
            }
            frame #4 {
              # "Vérifie que l'étoile de guidage s'est recentrée"
              n224 = local read "Undo offset"() -> (w403:bool)
              n225 = Not(x=w403) -> (.not. x?=w402:bool)
              n226 = And(x=w401, y=w402) -> (x .and. y?=w400:bool)
              n227 = case shown="True" w400 {
                tunnel: w399 -> [_ w408]
                tunnel: w398 -> [_ w407]
                frame False {
                }
                frame True {
                  n228 = global read "Globals.vi" "MaxIm.ICCDCamera"() -> (w404:refnum<k7>)
                  n229 = while {
                    tunnel: w404 -> [w421]
                    tunnel: w407 -> [w413]
                    tunnel: w408 -> [w415]
                    tunnel: [w410] -> w406
                    tunnel: [w409] -> w405
                    i -> [w419]
                    stop <- w417 stop-if-true
                    n230 = property class="ICCDCamera"(reference=w421) -> (reference out=w410:refnum<k7>, "GuiderXError"=w414:sgl, "GuiderYError"=w416:sgl)  [unwired: 1 in, 1 out]
                    n231 = Not Equal?(x=w413, y=w414) -> (x != y?=w412:bool)
                    n232 = Not Equal?(x=w416, y=w415) -> (x != y?=w411:bool)
                    n233 = Or(x=w412, y=w411) -> (x .or. y?=w409:bool)
                    n234 = Wait (ms)(milliseconds to wait=u32 100) -> ()  [unwired: 1 out]
                    n235 = call "max-iteration.vi"("i max"=300, "i act"=w419, "Valeur entrante"=w409) -> ("break ?"=w417:bool)
                  }
                  n236 = case shown="True" w405 {
                    tunnel: w406 -> [_ w422]
                    frame False {
                    }
                    frame True {
                      n237 = while {
                        tunnel: [w430] -> w423
                        tunnel: w422 -> [w429]
                        i -> [w438]
                        stop <- w439 stop-if-true
                        n238 = property class="ICCDCamera"(reference=w429) -> ("GuiderXError"=w432:sgl, "GuiderYError"=w431:sgl)  [unwired: 1 in, 2 out]
                        n239 = Not Equal To 0?(x=w432) -> (x != 0?=w435:bool)
                        n240 = Not Equal To 0?(x=w431) -> (x != 0?=w436:bool)
                        n241 = call-poly "Pytagore.vi"("D2"=w431, "D1"=w432) -> ("DT"=w442:dbl)
                        n242 = Greater?(x=w438, y=300) -> (0:w430:bool)
                        n243 = Less?(x=w442, y=3.0) -> (x < y?=w434:bool)
                        n244 = Compound Arithmetic op=AND(w434, w435, w436) -> (w433:bool)
                        n245 = Wait Until Next ms Multiple(millisecond multiple=u32 200 ("n millisecondes")) -> ()  [unwired: 1 out]
                        n246 = Or(x=w433, y=w430) -> (x .or. y?=w439:bool)
                      }
                      n247 = case shown="True" w423 {
                        frame False {
                        }
                        frame True {
                          n248 = Two Button Dialog(message="L'étoile de guidage ne semble pas s'être recentré", 1:"Ignorer" ("Nom du bouton V (\"OK\")"), 2:"Interrompre" ("Nom du bouton V (\"OK\")")) -> (T button?=w424:bool)
                          n249 = case shown="True" w424 {
                            selector: w424 -> [_ w428]
                            frame False {
                            }
                            frame True {
                              n250 = local write "Undo offset"(w428) -> ()
                            }
                          }
                        }
                      }
                    }
                  }
                }
              }
            }
          }
        }
      }
    }
    frame #3 {
      # "MicroOffset"
      n251 = local read "Undo offset"() -> (w446:bool)
      n252 = Not(x=w446) -> (.not. x?=w447:bool)
      n253 = local read "Moffset"() -> (w448:bool)
      n254 = And(x=w447, y=w448) -> (x .and. y?=w445:bool)
      n255 = case shown="True" w445 {
        tunnel: w444 -> [_ w450]
        tunnel: w443 -> [_ w449]
        frame False {
        }
        frame True {
          n256 = stacked-sequence {
            seq-local: [_ w454 _ _] -> [_ _ w484 w496]
            seq-local: [w451 _ _ _] -> [_ w453 _ w497]
            tunnel: w449 -> [_ w456 w485 _]
            tunnel: w450 -> [_ w455 w486 _]
            frame #0 {
              # "Vérifie que le guidage est en marche"
              n257 = local read "Guider was running"() -> (w451:bool)
              n258 = case shown="False" w451 {
                frame False {
                  n259 = One Button Dialog(message="Le guidage doit être démarrer \npour effectuer un micro-offset\ncommande annulée       ") -> ()  [unwired: 1 in, 1 out]
                }
                frame True {
                }
              }
            }
            frame #1 {
              # "Effectue le micro-offset"
              n260 = case shown="True" w453 {
                selector: w453 -> [w457 _]
                tunnel: w456 -> [_ w459]
                tunnel: w455 -> [_ w458]
                tunnel: [w457 w460] -> w454
                frame False {
                }
                frame True {
                  # "Déplacer la sonde\nle guidage bouge le télescope"
                  # "Déplacer la sonde"
                  n261 = global read "Globals.vi" "Position P"() -> (w461:i32)
                  n262 = global read "Globals.vi" "Position Z"() -> (w462:i32)
                  n263 = global write "Globals.vi" "CibleY"(w459) -> ()
                  n264 = global write "Globals.vi" "CibleX"(w458) -> ()
                  n265 = global write "Globals.vi" "Moniteur table"(TRUE ("Direction")) -> ()
                  n266 = local read "TableVisaNumber"() -> (w466:refnum<visa-resource-name>)
                  n267 = while {
                    tunnel: u32 500 ("goto accel") -> [w476]
                    tunnel: u32 500 ("goto lent") -> [w475]
                    tunnel: u32 5000 ("goto accel") -> [w474]
                    tunnel: w459 -> [w473]
                    tunnel: w458 -> [w472]
                    tunnel: w461 -> [w471]
                    tunnel: w462 -> [w470]
                    tunnel: w466 -> [w469]
                    tunnel: [w468] -> w460
                    i -> [w479]
                    stop <- w468 stop-if-true
                    n268 = call "GotoTables(aligned).vi"("High Speed"=w474, "Acceleration Time"=w475, "Low Speed"=w476, "VISA resource name"=w469, "Pulse P"=w471, "Pulse Z"=w470, "Pulse X"=w472, "Pulse Y"=w473) -> ("OK Done"=w480:bool)
                    n269 = call "max-iteration.vi"("i max"=10, "i act"=w479, "Valeur entrante"=w480) -> ("break ?"=w468:bool)
                    n270 = Wait Until Next ms Multiple(millisecond multiple=u32 200) -> ()  [unwired: 1 out]
                  }
                  n271 = case shown="False" w460 {
                    selector: w460 -> [w481 _]
                    frame False {
                      n272 = global write "Globals.vi" "Moniteur table"(w481) -> ()
                      n273 = One Button Dialog(message="ATTENTION!!\nLa commande de déplacement\ndes tables a échoué.\nVérifiez le contrôleur des tables", button name ("OK")="OK" ("nom du bouton (\"OK\")")) -> ()  [unwired: 1 out]
                    }
                    frame True {
                    }
                  }
                }
              }
            }
            frame #2 {
              n274 = case shown="True" w484 {
                tunnel: w486 -> [_ w487]
                tunnel: w485 -> [_ w488]
                frame False {
                }
                frame True {
                  n275 = while {
                    tunnel: w488 -> [_]
                    tunnel: w487 -> [_]
                    i -> [w492]
                    stop <- w490 continue-if-true
                    n276 = global read "Globals.vi" "Moniteur table"() -> (w491:bool)
                    n277 = call "max-iteration.vi"("i max"=150, "i act"=w492, "Valeur entrante"=w491) -> ("break ?"=w490:bool)
                    n278 = Wait Until Next ms Multiple(millisecond multiple=u32 200) -> ()  [unwired: 1 out]
                  }
                }
              }
            }
            frame #3 {
              # "Vérifie que l'étoile de guidage s'est recentrée"
              n279 = local read "Undo offset"() -> (w495:bool)
              n280 = Not(x=w495) -> (.not. x?=w494:bool)
              n281 = Compound Arithmetic op=AND(w494, w497, w496) -> (w498:bool)
              n282 = case shown="True" w498 {
                frame False {
                  n283 = local write "Undo offset"(TRUE) -> ()
                }
                frame True {
                  n284 = while {
                    tunnel: [w503] -> w500
                    i -> [w511]
                    stop <- w512 stop-if-true
                    # "tolérance à réajuster"
                    n285 = global read "Globals.vi" "MaxIm.ICCDCamera"() -> (w502:refnum<k7>)
                    n286 = property class="ICCDCamera"(reference=w502) -> ("GuiderXError"=w505:sgl, "GuiderYError"=w504:sgl)  [unwired: 1 in, 2 out]
                    n287 = Greater?(x=w511, y=300) -> (0:w503:bool)
                    n288 = Not Equal To 0?(x=w505) -> (x != 0?=w508:bool)
                    n289 = Not Equal To 0?(x=w504) -> (x != 0?=w509:bool)
                    n290 = call-poly "Pytagore.vi"("D2"=w504, "D1"=w505) -> ("DT"=w515:dbl)
                    n291 = Less?(x=w515, y=3.0) -> (x < y?=w507:bool)
                    n292 = Compound Arithmetic op=AND(w507, w508, w509) -> (w506:bool)
                    n293 = Or(x=w506, y=w503) -> (x .or. y?=w512:bool)
                    n294 = Wait Until Next ms Multiple(millisecond multiple=u32 200 ("n millisecondes")) -> ()  [unwired: 1 out]
                  }
                  n295 = case shown="True" w500 {
                    frame False {
                    }
                    frame True {
                      n296 = One Button Dialog(message="L'étoile de guidage ne semble pas s'être recentré") -> ()  [unwired: 1 in, 1 out]
                    }
                  }
                }
              }
            }
          }
        }
      }
    }
    frame #4 {
      # "Fermeture"
      n297 = global read "Globals.vi" "MaxIm.ICCDCamera"() -> (w518:refnum<k7>)
      n298 = property class="ICCDCamera"(reference=w518, "GuiderAggressivenessX"=w517, "GuiderAggressivenessY"=w516) -> ()  [unwired: 1 in, 2 out]
    }
  }
